vi "Cel_Faren.vi"() -> ()   [LabVIEW 2024]
panel:
  out "Numeric 2":dbl
  in  "Numeric":dbl
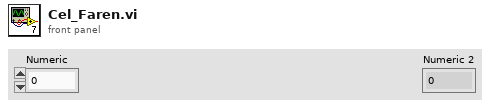
[diagram p1: front panel]
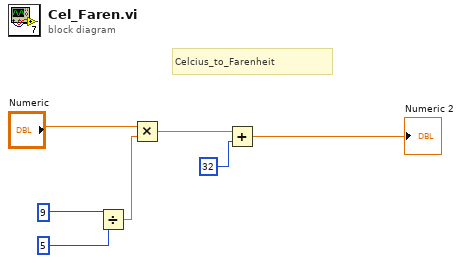
[diagram p0: block diagram]
diagram:
  # "Celcius_to_Farenheit"
  n1 = Divide(x=9, y=5) -> (x/y=w4:dbl)
  n2 = Multiply(x="Numeric", y=w4) -> (x*y=w2:dbl)
  n3 = Add(x=w2, y=32) -> (x+y=→"Numeric 2":dbl)
